vi "MakeWarning.vi"(0 "String":string, 2 "Enable":bool, 5 "Setup":u8=5, 11 "error in":errorcluster) -> (4 "Warning":bool, 15 "error out":errorcluster)   [LabVIEW 2011]
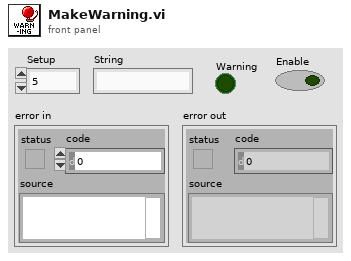
[diagram p1: front panel]
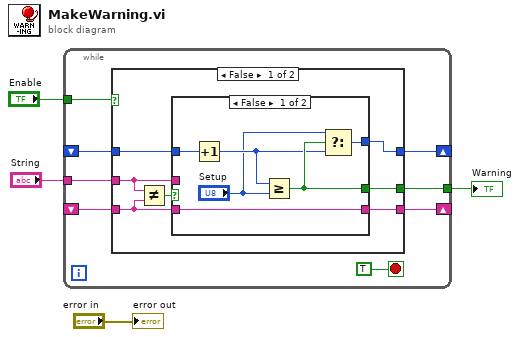
[diagram p0: block diagram]
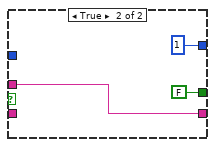
[diagram p2: hidden frame]
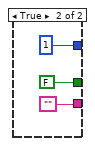
[diagram p3: hidden frame]
diagram:
  n1 = while {
    tunnel: "String" -> [w12]
    shift-right: [w11] -> _
    shift-left: _ -> [w10]
    shift-right: [w8] -> _
    shift-left: _ -> [w9]
    tunnel: [w6] -> w3
    tunnel: "Enable" -> [w5]
    stop <- TRUE stop-if-true
    n2 = case shown="False" w5 {
      tunnel: w12 -> [w19 _]
      tunnel: [w18 ""] -> w11
      tunnel: w10 -> [w17 _]
      tunnel: w9 -> [w16 _]
      tunnel: [w15 u8 1 ("Setup")] -> w8
      tunnel: [w14 FALSE] -> w6
      frame False {
        n3 = Not Equal?(x=w19, y=w17) -> (x != y?=w13:bool)
        n4 = case shown="False" w13 {
          tunnel: w19 -> [_ w28]
          tunnel: [w25 w28] -> w18
          tunnel: w17 -> [w25 _]
          tunnel: w16 -> [w24 _]
          tunnel: [w23 u8 1] -> w15
          tunnel: [w22 FALSE] -> w14
          frame False {
            n5 = Increment(x=w24) -> (x+1=w21:u8)
            n6 = Greater Or Equal?(x=w21, y="Setup") -> (x >= y?=w22:bool)
            n7 = Select(t="Setup", s=w22, f=w21) -> (s? t:f=w23:u8)
          }
          frame True {
          }
        }
      }
      frame True {
      }
    }
  }
  "Warning" <- w3
  "error out" <- "error in"
